vi "Delete.vi"(8 "error in (no error)":errorcluster, 10 "TopLevel In":T1, 11 "QSM In":string[](array[string])) -> (0 "error out":errorcluster, 2 "TopLevel Out":T1, 3 "QSM Out":string[](array[string]))   [LabVIEW 2011]
uses:
  Controls/Top Level Control.ctl
  <vilib>/NI/AMC/Message Queue.ctl
  <vilib>/NI/AMC/Message.ctl
  <vilib>/NI/Tools/Keyed Array/KeyedArray.ctl
  Controls/ListBox Test Record.ctl
  Controls/DVR of CSV Tests Data.ctl
  Controls/CSVs Tests Data.ctl
  Controls/Test Column Data.ctl
  Controls/Options DVR.ctl
  Controls/Options.ctl
  <userlib>/_OpenG.lib/array/array.llb/Delete Elements from Array__ogtk.vi
  <userlib>/_OpenG.lib/array/array.llb/Delete Elements from 1D Array (Path)__ogtk.vi
  <userlib>/_OpenG.lib/array/array.llb/Delete Elements from 1D Array (String)__ogtk.vi
  <vilib>/NI/Tools/Keyed Array/Tools_KeyedArray.lvlib
  <vilib>/NI/AMC/AMC.lvlib
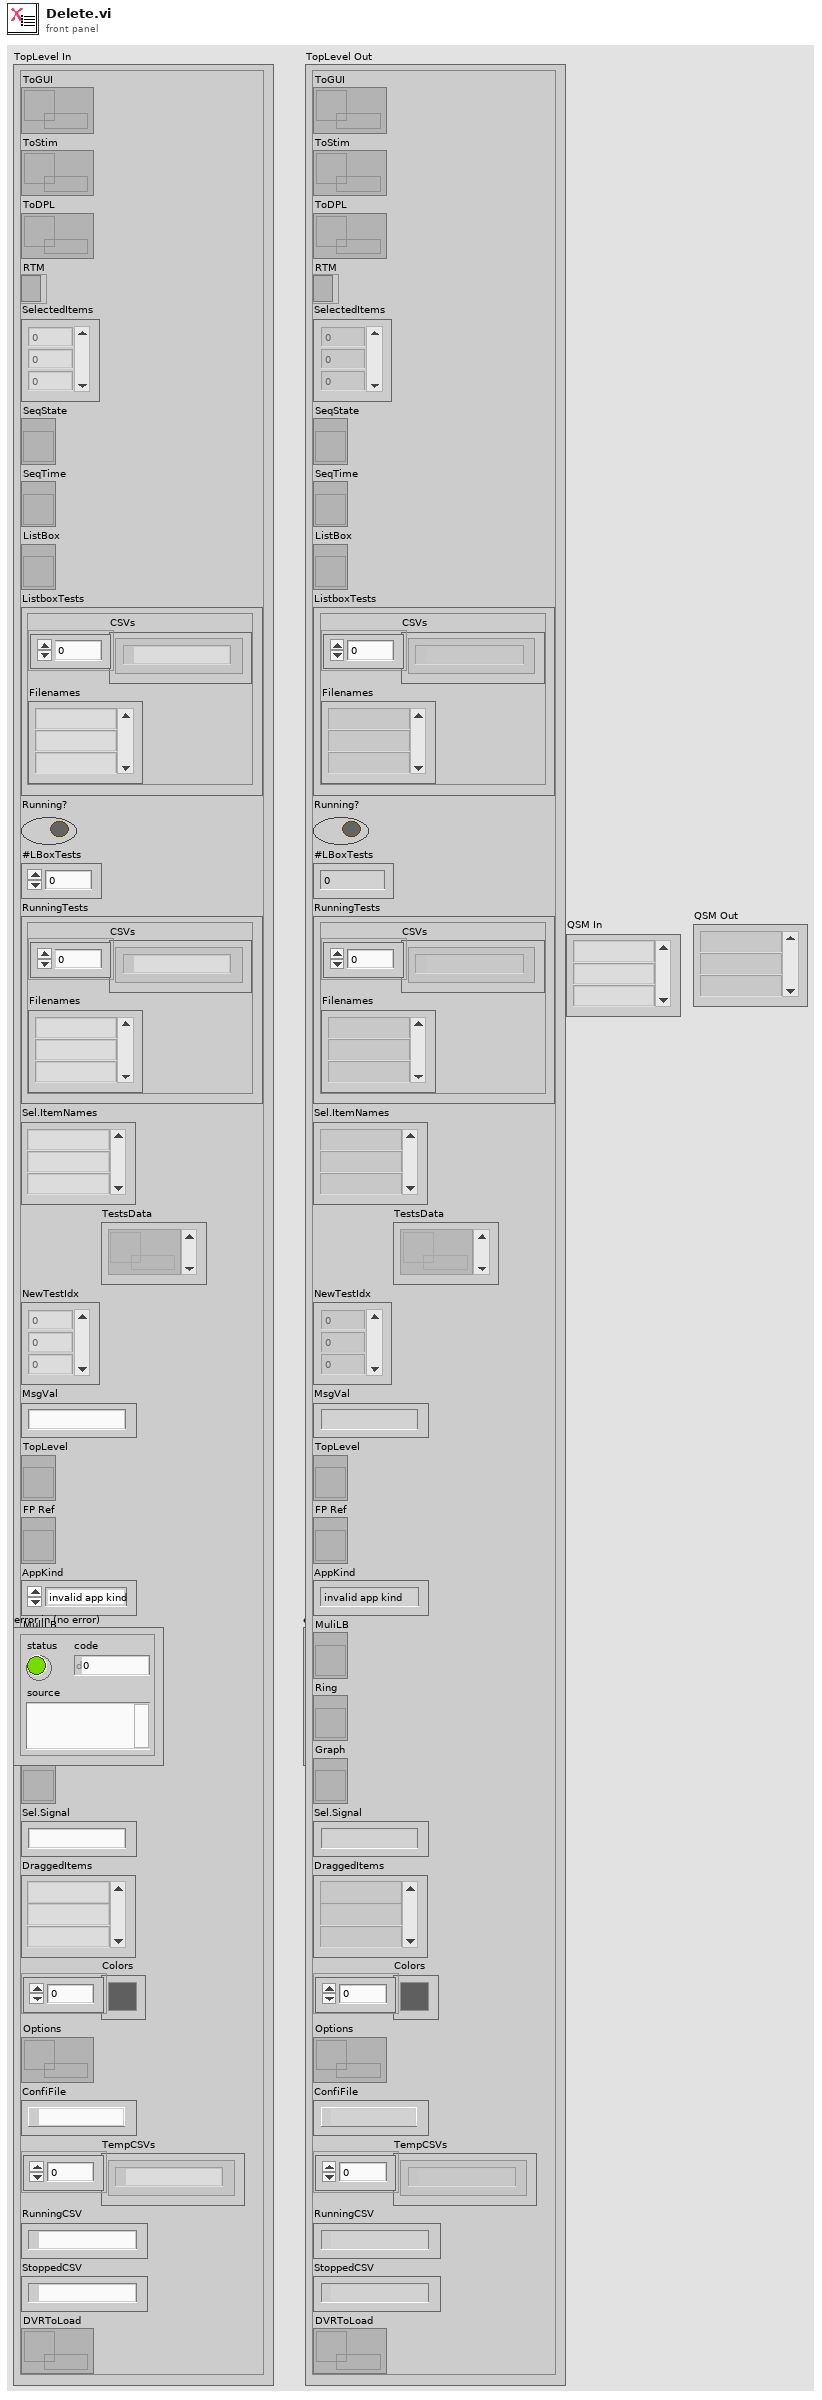
[diagram p1: front panel]
types:
  T1 = typedef "Top Level Control.ctl" = cluster{"ToGUI":T2, "ToStim":T2, "ToDPL":T2, "RTM":refnum<k9>, "SelectedItems":i32[], "SeqState":refnum<vi>, "SeqTime":refnum<vi>, "ListBox":refnum<vi>, "ListboxTests":T3, "Running?":bool, "#LBoxTests":i32, "RunningTests":T3, "Sel.ItemNames":string[], "TestsData":T4[], "NewTestIdx":i32[], "MsgVal":string, "TopLevel":refnum<vi>, "FP Ref":refnum<vi>, "AppKind":enum32{"invalid app kind", "Development System", "Run Time System", "Student Edition", "Embedded LabVIEW", "Evaluation", "Custom"}, "MuliLB":refnum<vi>, "Ring":refnum<vi>, "Graph":refnum<vi>, "Sel.Signal":string, "DraggedItems":string[], "Colors":u32[], "Options":T5, "ConfiFile":path, "TempCSVs":path[], "RunningCSV":path, "StoppedCSV":path, "DVRToLoad":T4}
  T2 = typedef "AMC.lvlib/Message Queue.ctl" = refnum<queue>
  T3 = typedef "ListBox Test Record.ctl" = cluster{"CSVs":path[], "Filenames":string[]}
  T4 = typedef "DVR of CSV Tests Data.ctl" = refnum<data-value>
  T5 = typedef "Options DVR.ctl" = refnum<data-value>
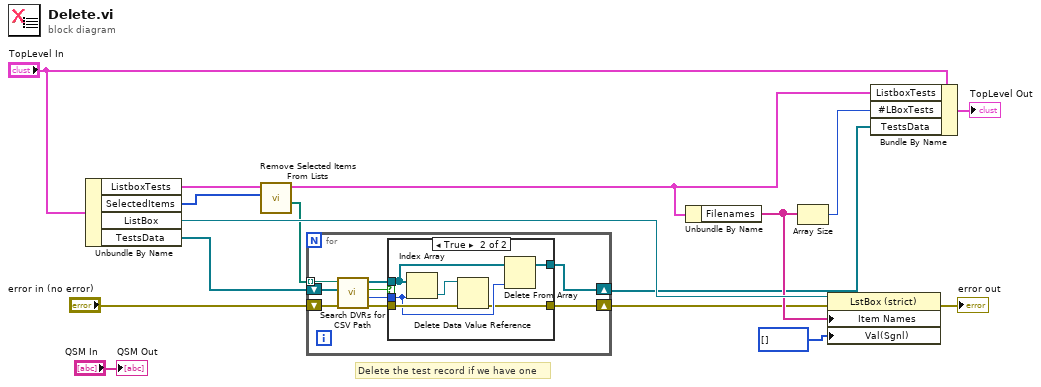
[diagram p0: block diagram]
diagram:
  # "Delete the test record if we have one"
  n1 = Unbundle By Name("TopLevel In") -> ("ListboxTests"=w11:T3, "SelectedItems"=w10:i32[], "ListBox"=w9:refnum<vi>, "TestsData"=w4:T4[])
  n2 = call "Remove Selected Items From Lists.vi"("SelectedItems"=w10, "ListBox Tests In"=w11) -> ("Deleted CSV(s)"=w3:path[], "ListBox Tests In Out"=w8:T3)  [unwired: 8 in]
  n3 = for {
    tunnel: w3 -> [w23] mode=indexing
    shift-right: [w18] -> w2
    shift-left: "error in (no error)" -> [w25]
    shift-right: [w17] -> w1
    shift-left: w4 -> [w24]
    n4 = call "Search DVRs for CSV Path.vi"("error in (no error)"=w25, "DVRs"=w24, "CsvPath"=w23) -> ("error out"=w19:errorcluster, "Idx"=w20:i32, "Found?"=w22:bool, "DVRs dup"=w21:T4[])  [unwired: 5 in]
    n5 = case shown="True" w22 {
      tunnel: w21 -> [w27 w31]
      tunnel: w20 -> [_ w30]
      tunnel: w19 -> [w26 w33]
      tunnel: [w26 w29] -> w18
      tunnel: [w27 w28] -> w17
      frame False {
      }
      frame True {
        n6 = Index Array(array=w31, index=w30) -> (element=w32:T4)
        n7 = Delete Data Value Reference(data value reference=w32, error in=w33) -> (error out=w29:errorcluster)  [unwired: 1 out]
        n8 = Delete From Array(array=w31, index=w30) -> (array with subset deleted=w28:T4[])  [unwired: 1 in, 1 out]
      }
    }
  }
  n9 = Unbundle By Name(w8) -> ("Filenames"=w7:string[])
  n10 = Array Size(array=w7) -> (size(s)=w6:i32)
  n11 = property on="Property Node" class="LstBox (strict)"(reference=w9, error in=w2, "Item Names"=w7, "Val(Sgnl)"=i32[] [] ("Tests")) -> (error out=→"error out":errorcluster)  [unwired: 1 out]
  n12 = Bundle By Name(cluster="TopLevel In", "ListboxTests"=w8, "#LBoxTests"=w6, "TestsData"=w1) -> (→"TopLevel Out":T1)
  "QSM Out" <- "QSM In"
